vi "zadanie_4.vi"() -> ()   [LabVIEW 2020]
panel:
  in  "Amplituda Y":dbl(slide) scale=0.0..10.0
  in  "Amplituda X":dbl(slide) scale=0.0..10.0
  in  "Częstotliwość Y":dbl(slide) scale=0.0..10.0
  in  "Częstotliwość X":dbl(slide) scale=0.0..10.0
  in  "Faza Y":dbl(slide) scale=0.0..180.0
  in  "Faza X":dbl(slide) scale=0.0..180.0
  out "XY Graph":cluster{"Y":dbl[], "Y":dbl[]}[](graph)
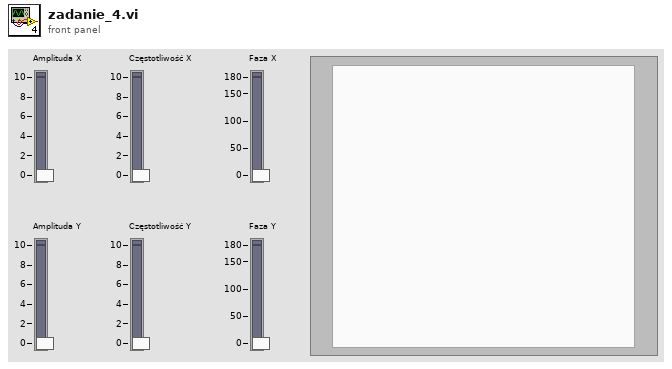
[diagram p1: front panel]
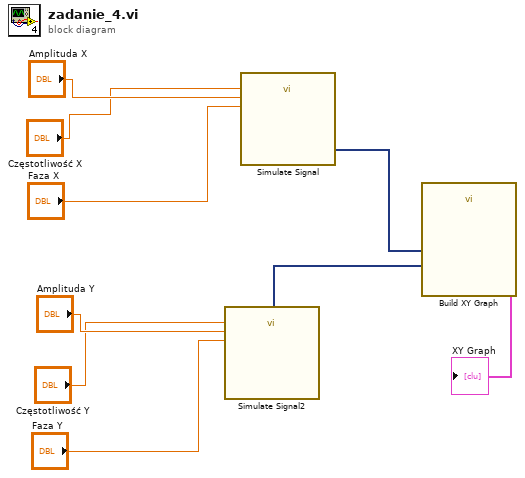
[diagram p0: block diagram]
diagram:
  n1 = call "Simulate Signal2"("Frequency"="Częstotliwość Y", "Amplitude"="Amplituda Y", "Phase"="Faza Y") -> ("Sine"=w6:dynamicdata)  [unwired: 11 in, 1 out]
  n2 = call "Simulate Signal"("Frequency"="Częstotliwość X", "Amplitude"="Amplituda X", "Phase"="Faza X") -> ("Sine"=w5:dynamicdata)  [unwired: 11 in, 1 out]
  n3 = call "Build XY Graph"("Y Input"=w6, "X Input"=w5) -> ("XY Graph"=→"XY Graph":cluster{"X":dbl[], "Y":dbl[]}[])  [unwired: 8 in, 1 out]
